vi "PathPlanner_FieldUtil_FlipFieldSpeeds.vi"(11 "FieldSpeeds":T1 {"vOmega" format="%10.3f"; "vY" format="%10.3f"; "vX" format="%10.3f"}) -> (3 "FlippedFieldSpeeds":T1 {"vOmega" format="%10.3f"; "vY" format="%10.3f"; "vX" format="%10.3f"})   [LabVIEW 2019, in "PathPlanner24.lvlib"]
doc: "Flip a field position\n\nInput:\n -- FieldPosition\n\nOutputs:\n -- FlippedFieldPosition"
uses:
  PathPlanner_FieldUtil_FieldSizeY.vi
  <vilib>/Rock Robotics/WPI/ThirdParty/JAS_Junk/TrajLib/Translation2d_GetXY.vi
  <vilib>/Rock Robotics/WPI/ThirdParty/JAS_Junk/TrajLib/Translation2d_Create.vi
  PathPlanner_FieldUtil_FieldSizeX.vi
  <vilib>/Rock Robotics/WPI/ThirdParty/JAS_Junk/TrajLib/Rotation2d_CreateAngle.vi
  <vilib>/Rock Robotics/WPI/ThirdParty/JAS_Junk/TrajLib/Rotation2d_Minus.vi
  <vilib>/Rock Robotics/WPI/ThirdParty/JAS_Junk/TrajLib/Conv_Feet_Meters.vi
  <vilib>/Rock Robotics/WPI/ThirdParty/JAS_Junk/TrajLib/Rotation2d_UnaryMinus.vi
  <vilib>/Rock Robotics/WPI/ThirdParty/JAS_Junk/TrajLib/Rotation2d_RotateBy.vi
  <vilib>/Rock Robotics/WPI/ThirdParty/JAS_Junk/TrajLib/Rotation2d_CreateXY.vi
  <vilib>/Rock Robotics/WPI/ThirdParty/JAS_Junk/TrajLib/Util_CalcDist.vi
  PathPlanner24.lvlib
  <vilib>/Rock Robotics/WPI/ThirdParty/JAS_Junk/TrajLib/TypeDef/CHASSIS_SPEEDS.ctl
  <vilib>/Rock Robotics/WPI/ThirdParty/JAS_Junk/TrajLib/Trajectory_Library.lvlib
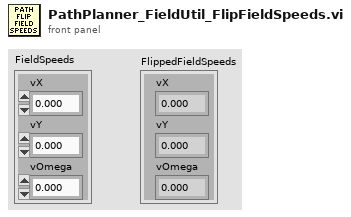
[diagram p1: front panel]
types:
  T1 = typedef "Trajectory_Library.lvlib/CHASSIS_SPEEDS.ctl" = cluster{"vX":dbl, "vY":dbl, "vOmega":dbl}
  T2 = typedef "PathPlanner24.lvlib/PathPlanner_FieldSymmetry_ENUM.ctl" = enum16{"kRotational", "kMirrored"}
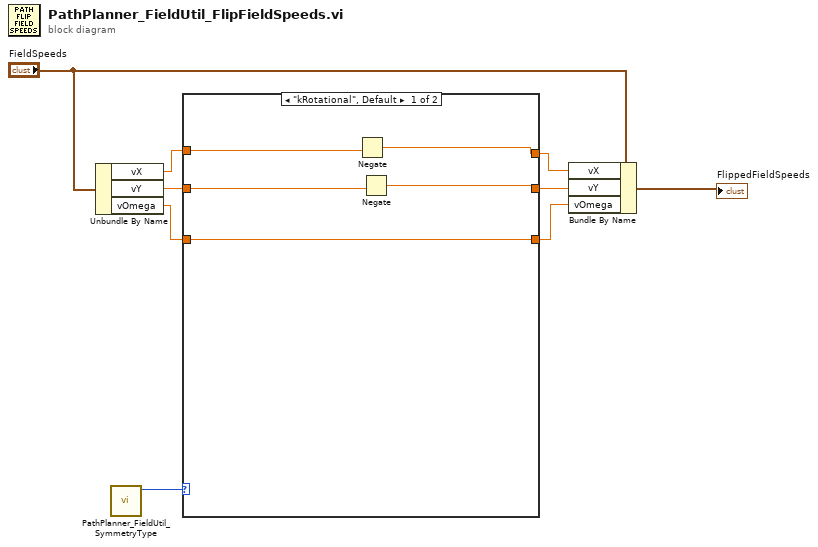
[diagram p0: block diagram]
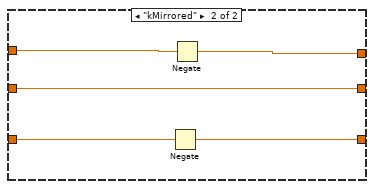
[diagram p2: hidden frame]
diagram:
  n1 = Unbundle By Name("FieldSpeeds") -> ("vX"=w6:dbl, "vY"=w4:dbl, "vOmega"=w2:dbl)
  n2 = call "PathPlanner_FieldUtil_SymmetryType.vi"() -> ("PathPlanner_FieldSymmetry"=w8:T2)  [unwired: 11 in]
  n3 = case shown="\"kRotational\", Default" w8 {
    tunnel: w6 -> [w14 w19]
    tunnel: [w11 w18] -> w5
    tunnel: w4 -> [w13 w17]
    tunnel: [w10 w17] -> w3
    tunnel: w2 -> [w12 w16]
    tunnel: [w12 w15] -> w1
    frame "kRotational", Default {
      n4 = Negate(x=w14) -> (-x=w11:dbl)
      n5 = Negate(x=w13) -> (-x=w10:dbl)
    }
    frame "kMirrored" {
      n6 = Negate(x=w16) -> (-x=w15:dbl)
      n7 = Negate(x=w19) -> (-x=w18:dbl)
    }
  }
  n8 = Bundle By Name(cluster="FieldSpeeds", "vX"=w5, "vY"=w3, "vOmega"=w1) -> (→"FlippedFieldSpeeds":T1)
